vi "RSZVB Trace Set RGB Color.vi"(0 "VISA session":refnum<visa-resource-name>, 1 "Trace Name (Trc1)":string="Trc1", 5 "Red (0)":dbl format="%^.3e", 7 "Green (0)":dbl format="%^.3e", 9 "Blue (0)":dbl format="%^.3e", 11 "error in (no error)":errorcluster {"code" format="%.0x"}, 12 "Trace Width (1)":i32=1, 13 "Trace Style (0: Solid)":i32(ring) items=["Solid", "Dashed", "Dotted", "DDotted", "DDDotted"]) -> (4 "dup VISA session":refnum<visa-resource-name>, 15 "error out":errorcluster {"code" format="%.0x"})   [LabVIEW 2011]
doc: "This VI defines the color of selected trace based on the Red/Green/Blue color model.\n\nRemote-control command(s):\nDISPlay:CMAP<13..28>:RGB <red>, <green>, <blue> ,<trace_style>, <trace_width>"
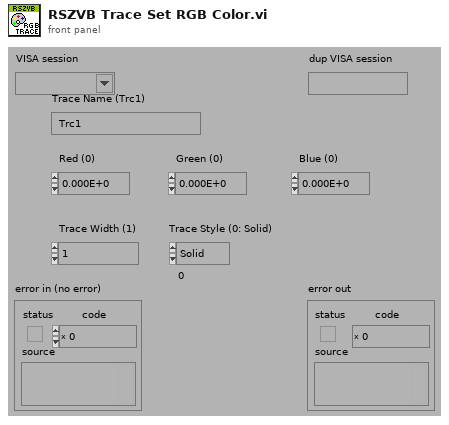
[diagram p1: front panel]
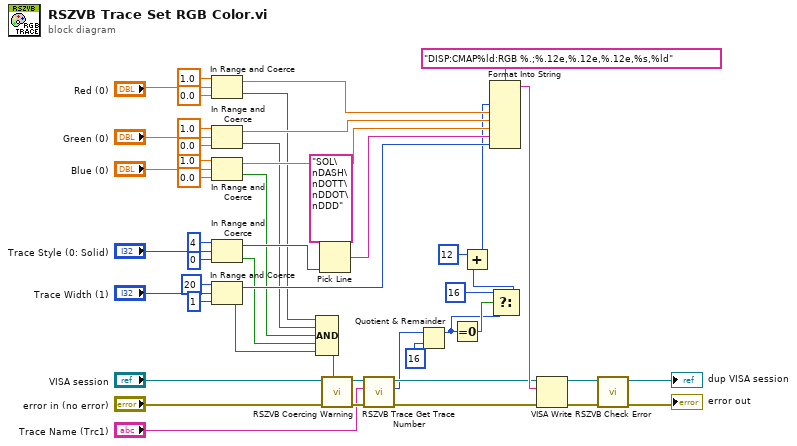
[diagram p0: block diagram]
diagram:
  n1 = In Range and Coerce(upper limit=1.0, x="Red (0)", lower limit=0.0) -> (coerced(x)=w36:dbl, In Range?=w29:bool)
  n2 = In Range and Coerce(upper limit=1.0, x="Green (0)", lower limit=0.0) -> (coerced(x)=w35:dbl, In Range?=w28:bool)
  n3 = In Range and Coerce(upper limit=1.0, x="Blue (0)", lower limit=0.0) -> (coerced(x)=w34:dbl, In Range?=w27:bool)
  n4 = In Range and Coerce(upper limit=4, x="Trace Style (0: Solid)", lower limit=0) -> (coerced(x)=w32:i32, In Range?=w26:bool)
  n5 = In Range and Coerce(upper limit=20, x="Trace Width (1)", lower limit=1) -> (coerced(x)=w30:i32, In Range?=w25:bool)
  n6 = Compound Arithmetic op=AND(w29, w28, w27, w26, w25) -> (w47:bool)
  n7 = Pick Line(multi-line string="SOL\nDASH\nDOTT\nDDOT\nDDD", line index=w32) -> (output string=w31:string)  [unwired: 1 in]
  n8 = call "RSZVB Coercing Warning.vi"("In Range?"=w47, "error in (no error)"="error in (no error)", "VISA session"="VISA session") -> ("error out"=w17:errorcluster, "dup VISA session"=w16:refnum<visa-resource-name>)  [unwired: 7 in]
  n9 = call "RSZVB Trace Get Trace Number.vi"("error in (no error)"=w17, "Trace Name (Trc1)"="Trace Name (Trc1)", "VISA session"=w16) -> ("error out"=w18:errorcluster, "Trace Number"=w2:i32, "dup VISA session"=w15:refnum<visa-resource-name>)  [unwired: 6 in]
  n10 = Quotient & Remainder(x=w2, y=16) -> (x-y*floor(x/y)=w1:i32)  [unwired: 1 out]
  n11 = Equal To 0?(x=w1) -> (x = 0?=w11:bool)
  n12 = Select(t=16 ("upper limit"), s=w11, f=w1) -> (s? t:f=w9:i32)
  n13 = Add(x=12, y=w9) -> (x+y=w5:i32)
  n14 = Format Into String(format string="DISP:CMAP%ld:RGB %.;%.12e,%.12e,%.12e,%s,%ld", w5, w36, w35, w34, w31, w30) -> (resulting string=w24:string)  [unwired: 2 in, 1 out]
  n15 = VISA Write(VISA resource name=w15, write buffer=w24, error in (no error)=w18) -> (VISA resource name out=w49:refnum<visa-resource-name>, error out=w48:errorcluster)  [unwired: 1 out]
  n16 = call "RSZVB Check Error.vi"("error in (no error)"=w48, "VISA session"=w49) -> ("error out"=→"error out":errorcluster, "dup VISA session"=→"dup VISA session":refnum<visa-resource-name>)  [unwired: 8 in]
